vi "Utility.FindNewDataFile.vi"(7 "Results Path":path=path "c:/testdata/temp", 8 "error in (no error)":errorcluster, 9 "LookupTable":variant, 10 "Remote Path":path=path "c:/testdata/temp", 11 "Path":path) -> (0 "error out":errorcluster, 1 "LookupTable out":variant, 2 "Found":bool, 3 "path out":path)   [LabVIEW 2014, in "NIAnalysis.lvlib"]
uses:
  NIAnalysis.lvlib
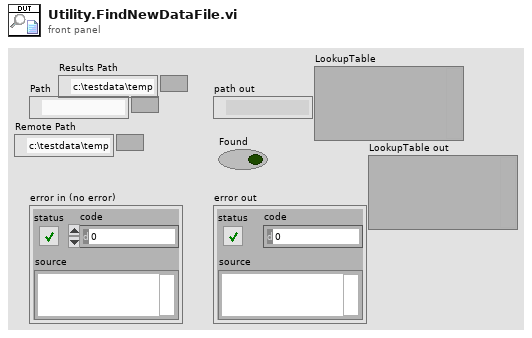
[diagram p1: front panel]
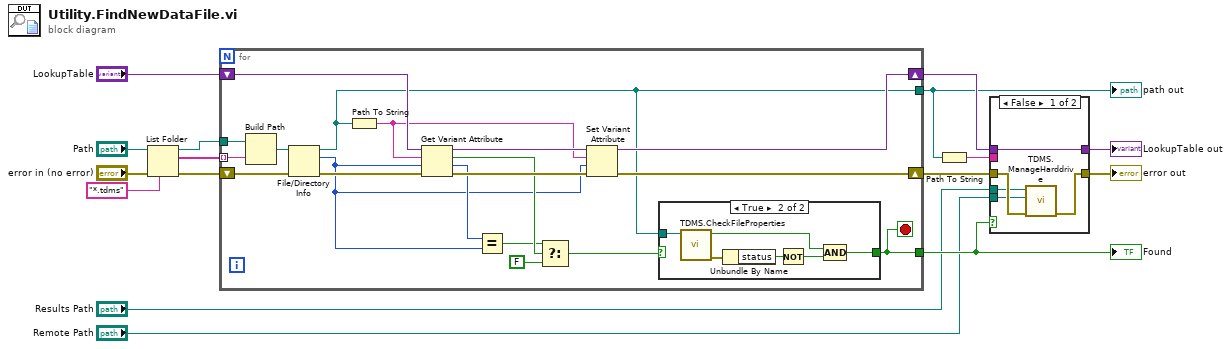
[diagram p0: block diagram]
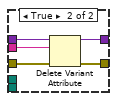
[diagram p2: hidden frame]
diagram:
  n1 = List Folder(path="Path", pattern="*.tdms", error in="error in (no error)") -> (path out=w12:path, filenames=w13:string[], error out=w14:errorcluster)  [unwired: 1 in, 1 out]
  n2 = for {
    tunnel: w12 -> [w35]
    tunnel: w13 -> [w34] mode=indexing
    shift-right: [w27] -> w9
    shift-left: w14 -> [w33]
    tunnel: [w17] -> w3
    tunnel: [w19] -> w4
    shift-right: [w20] -> w7
    shift-left: "LookupTable" -> [w30]
    stop <- w17 stop-if-true
    n3 = Build Path(base path=w35, name or relative path=w34) -> (appended path=w32:path)
    n4 = File/Directory Info(path=w32, error in=w33) -> (path out=w19:path, size=w23:i64, error out=w31:errorcluster)  [unwired: 4 out]
    n5 = Path To String(path=w19) -> (string=w26:string)
    n6 = Get Variant Attribute(Variant=w30, name=w26, default value (empty Variant)=w23, error in=w31) -> (duplicate Variant=w29:variant, found=w25:bool, value=w24:i64, error out=w28:errorcluster)
    n7 = Equal?(x=w24, y=w23) -> (x = y?=w22:bool)
    n8 = Select(t=w22, s=w25, f=FALSE) -> (s? t:f=w18:bool)
    n9 = Set Variant Attribute(Variant=w29, name=w26, value=w23, error in=w28) -> (Variant out=w20:variant, error out=w27:errorcluster)  [unwired: 1 out]
    n10 = case shown="True" w18 {
      selector: w18 -> [w36 _]
      tunnel: w19 -> [_ w40]
      tunnel: [w36 w38] -> w17
      frame False {
      }
      frame True {
        n11 = call "TDMS.CheckFileProperties.vi"("Data"=w40) -> ("error out"=w39:errorcluster, "Found All"=w37:bool)  [unwired: 9 in]
        n12 = Unbundle By Name(w39) -> ("status"=w42:bool)
        n13 = Not(x=w42) -> (.not. x?=w41:bool)
        n14 = Compound Arithmetic op=AND(w37, w41) -> (w38:bool)
      }
    }
  }
  "path out" <- w4
  "Found" <- w3
  n15 = Path To String(path=w4) -> (string=w5:string)
  n16 = case shown="False" w3 {
    tunnel: w9 -> [w46 w52]
    tunnel: [w45 w51] -> w8
    tunnel: w7 -> [w47 w50]
    tunnel: [w47 w49] -> w6
    tunnel: w5 -> [_ w48]
    tunnel: "Results Path" -> [w44 _]
    tunnel: "Remote Path" -> [w43 _]
    frame False {
      n17 = call "TDMS.ManageHarddrive.vi"("error in"=w46, "Remote Path"=w43, "Results Path"=w44) -> ("error out"=w45:errorcluster)  [unwired: 8 in]
    }
    frame True {
      n18 = Delete Variant Attribute(4:w52, 6:w48, 7:w50) -> (0:w51:errorcluster, 3:w49:variant)  [unwired: 1 out]
    }
  }
  "error out" <- w8
  "LookupTable out" <- w6
